vi "compress_alarms.vi"(6 "N alr":i32, 9 "ALR state":T1(array[cluster]), 10 "time stamp":timestamp, 11 "table":string) -> (3 "parameters":string)   [LabVIEW 2019, in "PostgreSQL.lvlib"]
uses:
  PostgreSQL.lvlib
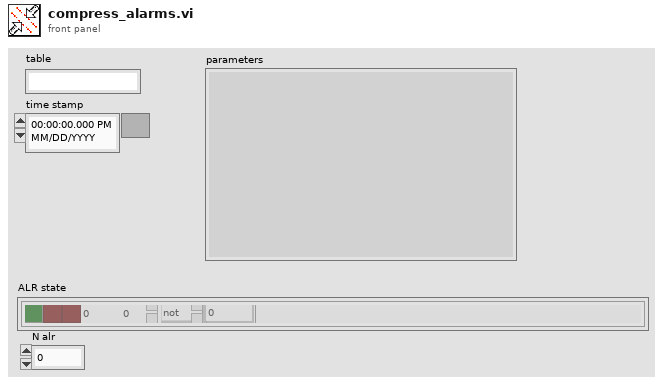
[diagram p1: front panel]
types:
  T1 = cluster{"ALR":bool, "ALR NOT block":bool, "ALR ON":bool, "t ms":u32, "alrnum":i32, "ack state":enum32{"not", "tripped", "reset", "ack"}, "color":u32, "alrname":string}[]
  T2 = cluster{"ALR":bool, "ALR NOT block":bool, "ALR ON":bool, "t ms":u32, "alrnum":i32, "ack state":enum32{"not", "tripped", "reset", "ack"}, "color":u32, "alrname":string}
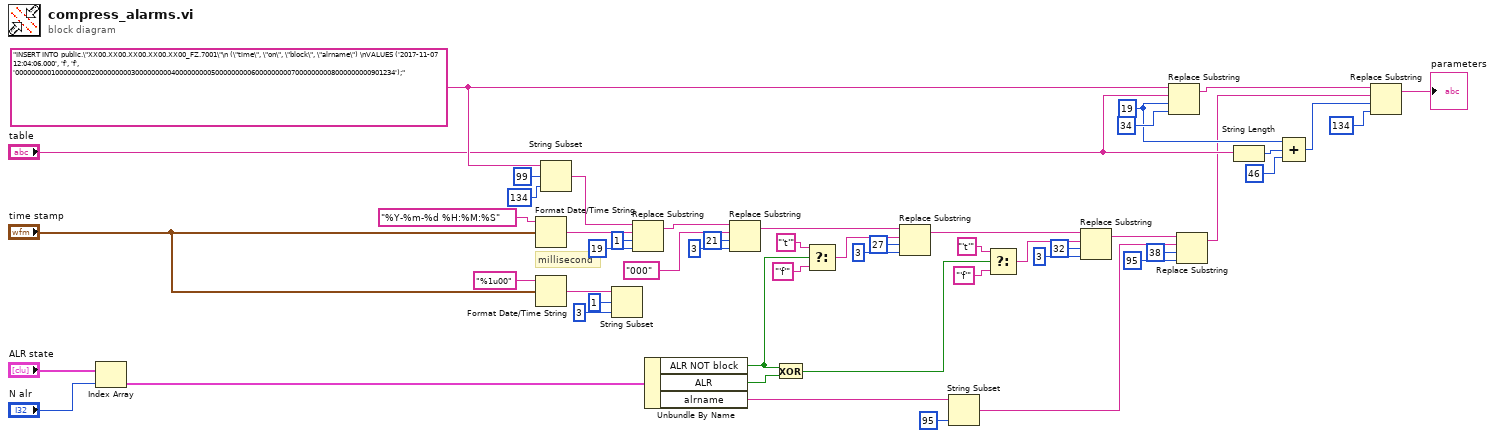
[diagram p0: block diagram]
diagram:
  w29 = 19 ("offset (0)")
  w31 = "INSERT INTO public.\"XX00.XX00.XX00.XX00.XX00_FZ.7001\"\n (\"time\", \"on\", \"block\", \"alrname\") \nVALUES ('2017-11-07 12:04:06.000', 'f', 'f', '00000000010000000002000000000300000000040000000005000000000600000000070000000008000000000901234');" ("object 3")
  # "millisecond"
  n1 = Index Array(array="ALR state", index="N alr") -> (element=w24:T2)
  n2 = Format Date/Time String(time format string (%c)="%Y-%m-%d %H:%M:%S", seconds (now)="time stamp") -> (date/time string=w46:string)  [unwired: 1 in]
  n3 = Format Date/Time String(time format string (%c)="%1u00", seconds (now)="time stamp") -> (date/time string=w49:string)  [unwired: 1 in]
  n4 = String Subset(string=w31, offset (0)=99, length (rest)=134 ("length (rest)")) -> (substring=w30:string)
  n5 = String Subset(string=w49, offset (0)=1, length (rest)=3 ("length (rest)")) -> ()  [unwired: 1 out]
  n6 = Replace Substring(2:19 ("length (len. of substring)"), 3:1 ("offset (0)"), 4:w46, 5:w30) -> (1:w43:string)  [unwired: 1 out]
  n7 = Unbundle By Name(w24) -> ("ALR NOT block"=w1:bool, "ALR"=w15:bool, "alrname"=w13:string)
  n8 = Replace Substring(2:3 ("length (len. of substring)"), 3:21 ("offset (0)"), 4:"000", 5:w43) -> (1:w3:string)  [unwired: 1 out]
  n9 = Exclusive Or(1:w15, 2:w1) -> (0:w14:bool)
  n10 = Select(t="'t'", s=w1, f="'f'") -> (s? t:f=w5:string)
  n11 = Replace Substring(2:3 ("x+y"), 3:27 ("offset (0)"), 4:w5, 5:w3) -> (1:w2:string)  [unwired: 1 out]
  n12 = String Subset(string=w13, length (rest)=95 ("length (rest)")) -> (substring=w12:string)  [unwired: 1 in]
  n13 = Select(t="'t'", s=w14, f="'f'") -> (s? t:f=w21:string)
  n14 = Replace Substring(2:3 ("x+y"), 3:32 ("offset (0)"), 4:w21, 5:w2) -> (1:w16:string)  [unwired: 1 out]
  n15 = Replace Substring(2:34 ("length (len. of substring)"), 3:w29, 4:"table", 5:w31) -> (1:w28:string)  [unwired: 1 out]
  n16 = Replace Substring(2:95 ("x+y"), 3:38 ("offset (0)"), 4:w12, 5:w16) -> (1:w17:string)  [unwired: 1 out]
  n17 = String Length(string="table") -> (length=w37:i32)
  n18 = Compound Arithmetic op=ADD(w29, w37, 46 ("value")) -> (w35:i32)
  n19 = Replace Substring(2:134 ("length (len. of substring)"), 3:w35, 4:w17, 5:w28) -> (1:→"parameters":string)  [unwired: 1 out]
